vi "Stop Do.vi"(8 "error in (no error)":errorcluster, 11 "ITask Actor in":refnum<class "ITask Actor.lvclass">) -> (0 "error out":errorcluster, 3 "ITask Actor out":refnum<class "ITask Actor.lvclass">)   [LabVIEW 2023, in "HAL GOOP4.lvlib" / "ITask Actor.lvlib" / "ITask Actor.lvclass"]
uses:
  ITask Actor.lvclass
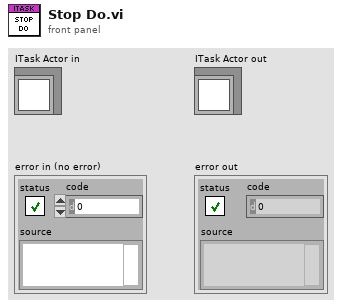
[diagram p1: front panel]
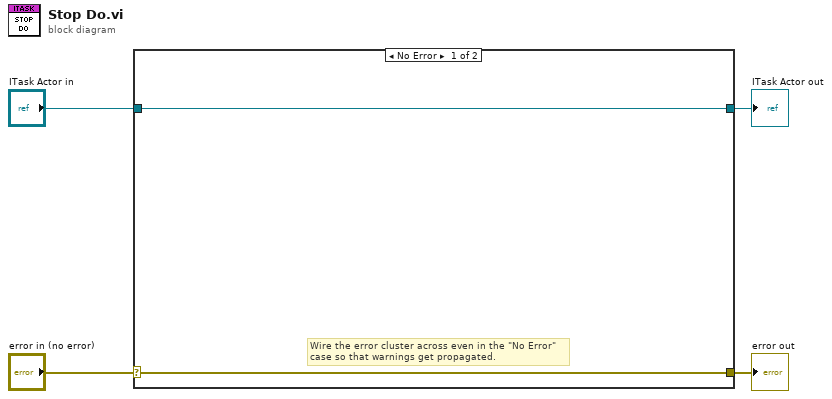
[diagram p0: block diagram]
diagram:
  n1 = case shown="No Error" "error in (no error)" {
    selector: "error in (no error)" -> [w5 w8]
    tunnel: [w5 w8] -> w3
    tunnel: [w6 w7] -> w1
    tunnel: "ITask Actor in" -> [w6 w7]
    frame No Error {
      # "Wire the error cluster across even in the \"No Error\"\ncase so that warnings get propagated."
    }
    frame Error {
    }
  }
  "error out" <- w3
  "ITask Actor out" <- w1
